vi "TDMS chan to HDF5 (bool).vi"(0 "tdms file":refnum<k34>, 1 "close dataset? (T)":bool=TRUE, 5 "group name in":string, 7 "channel name in":string, 11 "error in (no error)":errorcluster, 13 "HDF5 Ref":T1) -> (4 "tdms file out":refnum<k34>, 6 "group name out":string, 8 "channel name out":string, 10 "dataset out":T1, 15 "error out":errorcluster)   [LabVIEW 2012]
uses:
  <vilib>/addons/_hdf5/library.llb/HDF5 Ref.ctl
  <vilib>/addons/_hdf5/dataspace.llb/H5S_seloper_t.ctl
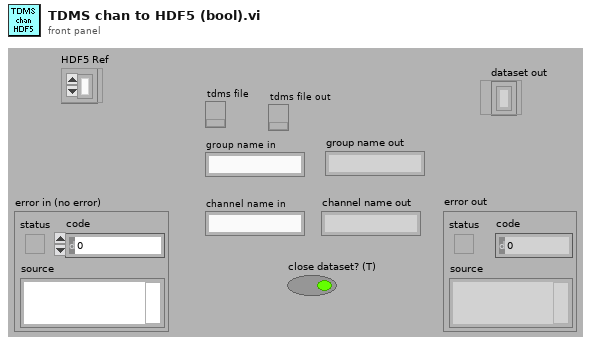
[diagram p1: front panel]
types:
  T1 = typedef "HDF5 Ref.ctl" = refnum<k1>
  T2 = typedef "H5S_seloper_t.ctl" = i32
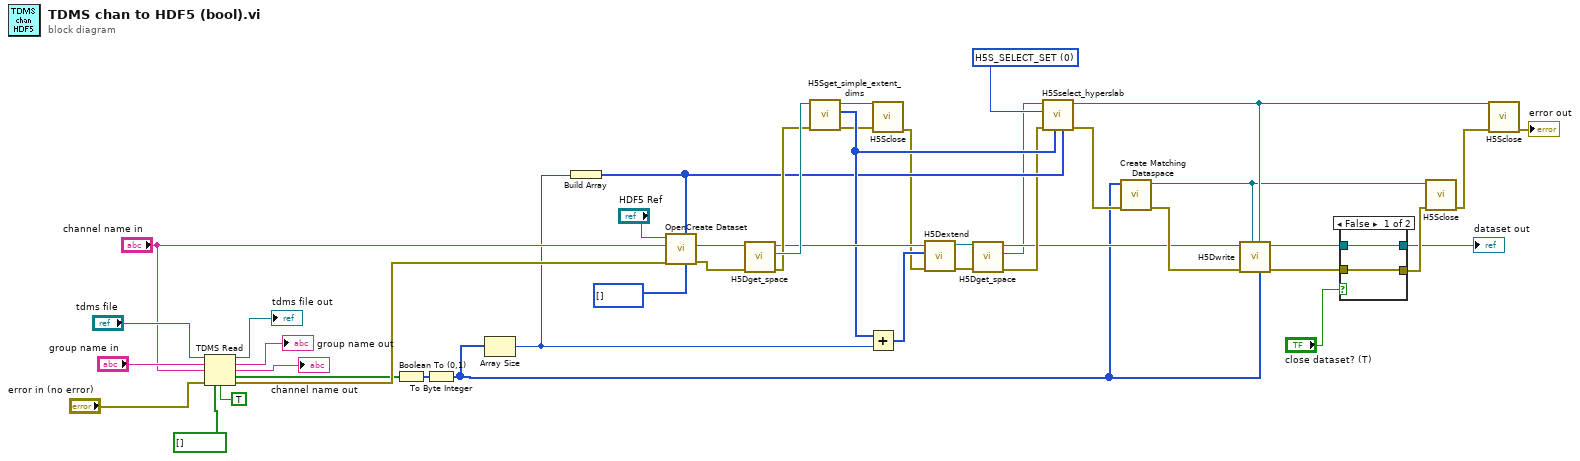
[diagram p0: block diagram]
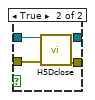
[diagram p2: hidden frame]
diagram:
  w33 = T2 0 items=["H5S_SELECT_NOOP"=-1, "H5S_SELECT_SET"=0, "H5S_SELECT_OR"=1, "H5S_SELECT_AND"=2, "H5S_SELECT_XOR"=3, "H5S_SELECT_NOTB"=4, "H5S_SELECT_NOTA"=5, "H5S_SELECT_APPEND"=6, "H5S_SELECT_PREPEND"=7] ("Operator")
  n1 = TDMS Read(0:"tdms file", 5:"group name in", 7:"channel name in", 11:"error in (no error)", 12:bool[] [], 13:TRUE ("return channels in file order? (F)")) -> (4:→"tdms file out":refnum<k34>, 6:→"group name out":string, 8:→"channel name out":string, 10:w5:bool[], 15:w39:errorcluster)  [unwired: 2 in, 1 out]
  n2 = Boolean To (0,1)(Boolean=w5) -> (0, 1=w3:i16[])
  n3 = To Byte Integer(number=w3) -> (8bit integer=w1:i8[])
  n4 = Array Size(array=w1) -> (size(s)=w19:i32)
  n5 = Build Array(w19) -> (w18:i32[])
  n6 = call "OpenCreate Dataset.vi"("Datatype"=i8[] [] ("0, 1"), "Chunk size"=w18, "error in (no error)"=w39, "Dataset Path"="channel name in", "HDF5 Ref"="HDF5 Ref") -> ("error out"=w38:errorcluster, "HDF5 Dataset Ref out"=w30:T1)  [unwired: 4 in, 1 out]
  n7 = call <vilib>:"H5Dget_space.vi"("error in (no error)"=w38, "HDF5 Dataset Ref"=w30) -> ("error out"=w36:errorcluster, "HDF5 Dataspace Ref"=w37:T1, "HDF5 Dataset Ref out"=w34:T1)  [unwired: 5 in]
  n8 = call <vilib>:"H5Sget_simple_extent_dims.vi"("error in (no error)"=w36, "HDF5 Space Ref"=w37) -> ("error out"=w17:errorcluster, "Dims"=w32:i32[], "HDF5 Ref out"=w16:T1)  [unwired: 4 in, 1 out]
  n9 = Add(x=w32, y=w19) -> (x+y=w35:i32[])
  n10 = call <vilib>:"H5Sclose.vi"("error in (no error)"=w17, "HDF5 Dataspace Ref"=w16) -> ("error out"=w13:errorcluster)  [unwired: 7 in]
  n11 = call <vilib>:"H5Dextend.vi"("error in (no error)"=w13, "Size"=w35, "HDF5 Dataset Ref"=w34) -> ("error out"=w14:errorcluster, "HDF5 Dataset Ref out"=w15:T1)  [unwired: 5 in]
  n12 = call <vilib>:"H5Dget_space.vi"("error in (no error)"=w14, "HDF5 Dataset Ref"=w15) -> ("error out"=w12:errorcluster, "HDF5 Dataspace Ref"=w10:T1, "HDF5 Dataset Ref out"=w11:T1)  [unwired: 5 in]
  n13 = call <vilib>:"H5Sselect_hyperslab.vi"("Count"=w18, "Start"=w32, "error in (no error)"=w12, "Operator"=w33, "HDF5 Space Ref"=w10) -> ("error out"=w31:errorcluster, "HDF5 Ref out"=w26:T1)  [unwired: 5 in]
  n14 = call <vilib>:"Create Matching Dataspace.vi"("error in (no error)"=w31, "Data"=w1) -> ("error out"=w29:errorcluster, "HDF5 Dataspace Ref"=w25:T1)  [unwired: 6 in]
  n15 = call <vilib>:"H5Dwrite.vi"("Variant"=w1, "HDF5 File Space Ref (H5S_ALL)"=w26, "HDF5 Memory Space Ref (H5S_ALL)"=w25, "error in (no error)"=w29, "HDF5 Dataset Ref"=w11) -> ("error out"=w27:errorcluster, "HDF5 Ref out"=w28:T1)  [unwired: 5 in]
  n16 = case shown="False" "close dataset? (T)" {
    tunnel: w28 -> [w46 w49]
    tunnel: w27 -> [w45 w48]
    tunnel: [w45 w47] -> w24
    tunnel: [w46 _] -> w6
    frame False {
    }
    frame True {
      n17 = call <vilib>:"H5Dclose.vi"("error in (no error)"=w48, "HDF5 Dataset Ref"=w49) -> ("error out"=w47:errorcluster)  [unwired: 7 in]
    }
  }
  "dataset out" <- w6
  n18 = call <vilib>:"H5Sclose.vi"("error in (no error)"=w24, "HDF5 Dataspace Ref"=w25) -> ("error out"=w23:errorcluster)  [unwired: 7 in]
  n19 = call <vilib>:"H5Sclose.vi"("error in (no error)"=w23, "HDF5 Dataspace Ref"=w26) -> ("error out"=→"error out":errorcluster)  [unwired: 7 in]
